vi "ChangeShutter.vi"(11 "Topas":refnum<k24>) -> (3 "Topas Out":refnum<k24>)   [LabVIEW 2017]
doc: "Shows how to open/close shutter and get current state."
uses:
  D:/upwork/Laser Measurement Tool/Topas4PublicAPI/NET_SDK/Topas4Lib.dll
  Topas4PublicAPI/NET_SDK/Topas4Lib.dll
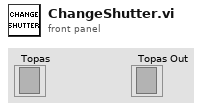
[diagram p1: front panel]
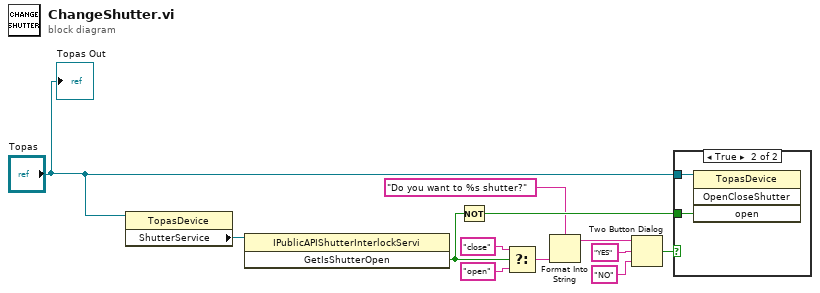
[diagram p0: block diagram]
diagram:
  n1 = property class="TopasDevice"(reference="Topas") -> ("ShutterService"=w11:refnum<k24>)  [unwired: 1 in, 2 out]
  n2 = invoke class="IPublicAPIShutterInterlockServi" method="GetIsShutterOpen"(reference=w11) -> ("GetIsShutterOpen"=w5:bool)  [unwired: 2 in, 2 out]
  n3 = Not(x=w5) -> (.not. x?=w10:bool)
  n4 = Select(t="close", s=w5, f="open") -> (s? t:f=w6:string)
  n5 = Format Into String(format string="Do you want to %s shutter?" ("message"), w6) -> (resulting string=w2:string)  [unwired: 2 in, 1 out]
  n6 = Two Button Dialog(message=w2, 1:"NO" ("F button name (\"Cancel\")"), 2:"YES" ("T button name (\"OK\")")) -> (T button?=w1:bool)
  n7 = case shown="True" w1 {
    tunnel: "Topas" -> [_ w14]
    tunnel: w10 -> [_ w13]
    frame False {
    }
    frame True {
      n8 = invoke class="TopasDevice" method="OpenCloseShutter"(reference=w14, "open"=w13) -> ()  [unwired: 2 in, 4 out]
    }
  }
  "Topas Out" <- "Topas"
